vi "runTemperatureAnalysis.vi"(8 "error in (no error)":errorcluster, 11 "ImageStreamViewer in":refnum<class "ImageStreamViewer.lvclass">) -> (0 "error out":errorcluster, 3 "ImageStreamViewer out":refnum<class "ImageStreamViewer.lvclass">)   [LabVIEW 2011, in "Views.lvlib" / "Camera.lvlib" / "ImageStreamViewer.lvclass"]
uses:
  ImageStreamViewer.lvclass
  Tools/ImageProcessor/ImageAnalyser/TemperatureAnalyser/TemperatureAnalyser.lvclass
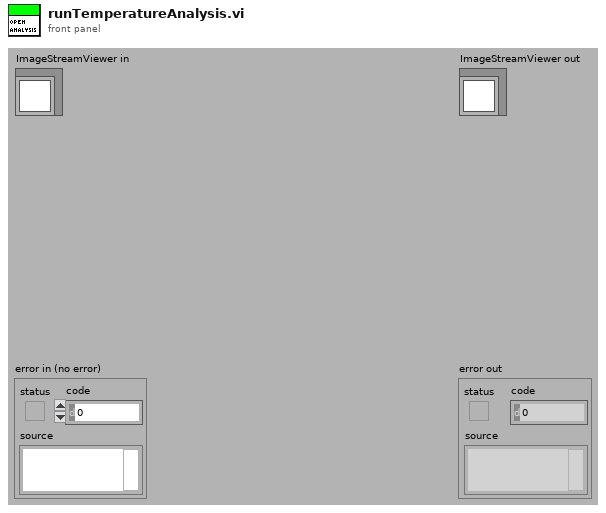
[diagram p1: front panel]
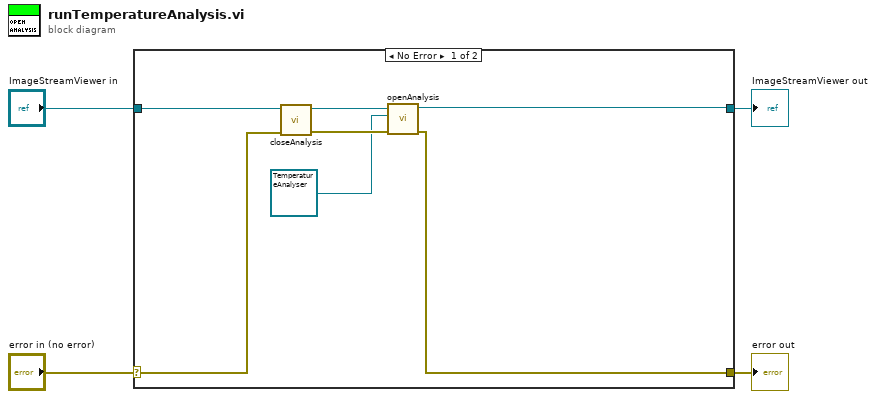
[diagram p0: block diagram]
diagram:
  n1 = case shown="No Error" "error in (no error)" {
    selector: "error in (no error)" -> [w6 w13]
    tunnel: [w10 w13] -> w3
    tunnel: [w11 w12] -> w1
    tunnel: "ImageStreamViewer in" -> [w9 w12]
    frame No Error {
      n2 = call "closeAnalysis.vi"("error in (no error)"=w6, "ImageStreamViewer in"=w9) -> ("error out"=w7:errorcluster, "ImageStreamViewer out"=w8:refnum<class "ImageStreamViewer.lvclass">)  [unwired: 8 in]
      n3 = call "openAnalysis.vi"("error in (no error)"=w7, "ImageAnalyser"=refnum<class "TemperatureAnalyser.lvclass"> refnum ("Tools.lvlib:Imaging.lvlib:TemperatureAnalyser.lvclass"), "ImageStreamViewer in"=w8) -> ("error out"=w10:errorcluster, "ImageStreamViewer out"=w11:refnum<class "ImageStreamViewer.lvclass">)  [unwired: 7 in]
    }
    frame Error {
    }
  }
  "error out" <- w3
  "ImageStreamViewer out" <- w1
